vi "ThisIsATest_II.vi"() -> ()   [LabVIEW 2016]
panel:
  out "everything is okay":bool
  in  "armed":bool
  out "wait timer 2":dbl
  out "wait timer":dbl
  in  "stop":bool
  out "Loop":dbl
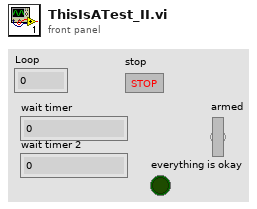
[diagram p1: front panel]
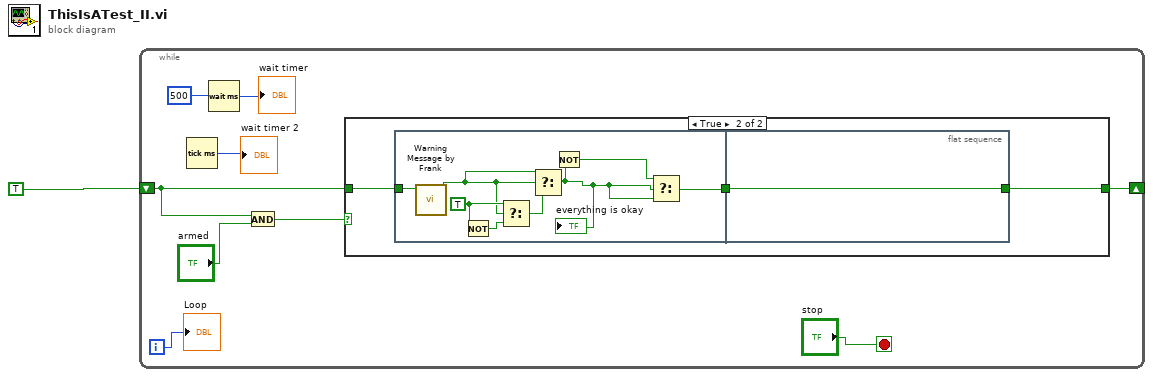
[diagram p0: block diagram]
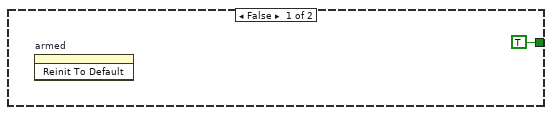
[diagram p2: hidden frame]
diagram:
  n1 = while {
    shift-right: [w5] -> _
    shift-left: TRUE ("Everything IS OK!") -> [w4]
    i -> [w10]
    stop <- "stop" stop-if-true
    n2 = Tick Count (ms)() -> (millisecond timer value=→"wait timer 2":u32)
    n3 = Wait (ms)(milliseconds to wait=500) -> (millisecond timer value=→"wait timer":u32)
    n4 = And(x=w4, y="armed") -> (x .and. y?=w2:bool)
    n5 = case shown="True" w2 {
      tunnel: [TRUE w14] -> w5
      tunnel: w4 -> [_ w12]
      frame False {
        n6 = invoke on="armed" class="Bool (strict)" method="Reinit To Default"() -> ()  [unwired: 3 in, 3 out]
      }
      frame True {
        n7 = flat-sequence {
          tunnel: [w17] -> w13
          tunnel: w12 -> [w22]
          tunnel: [w23] -> w14
          tunnel: w13 -> [w23]
          frame #0 {
            w21 = TRUE
            n8 = call "Warning Message by Frank.vi"("Arm Flag"=w22) -> ("super ok"=w18:bool)  [unwired: 8 in, 2 out]
            n9 = Not(x=w21) -> (.not. x?=w20:bool)
            n10 = Select(t=w21, s=w18, f=w20) -> (s? t:f=w19:bool)
            n11 = Select(t=w18, s=w18, f=w19) -> (s? t:f=w15:bool)
            "everything is okay" <- w15
            n12 = Not(x=w15) -> (.not. x?=w16:bool)
            n13 = Select(t=w16, s=w15, f=w15) -> (s? t:f=w17:bool)
          }
          frame #1 {
          }
        }
      }
    }
    "Loop" <- w10
  }
